vi "InterpretKeyboardCommand.vi"(6 "Key\nValue":i32, 8 "X Decreasing":string(combo)="10", 9 "X Increasing":string(combo)="13", 10 "Y Decreasing":string(combo)="28", 11 "Y Increasing":string(combo)="32") -> (0 "X Decreasing (#)":i32, 1 "X Increasing (#)":i32, 2 "Y Decreasing (#)":i32, 3 "Y Increasing (#)":i32, 4 "number":u32, 5 "Cluster of Input #s":cluster{i32, i32, i32, i32})   [LabVIEW 2011]
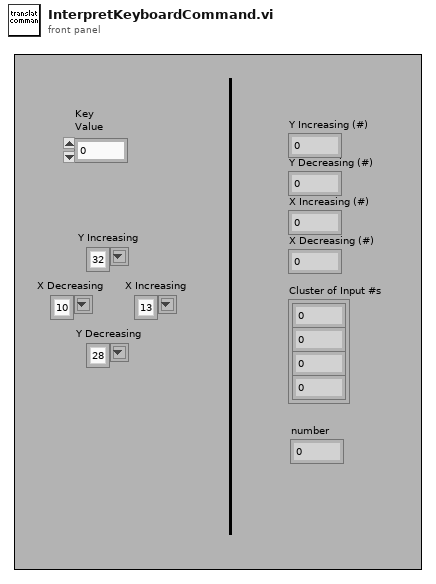
[diagram p1: front panel]
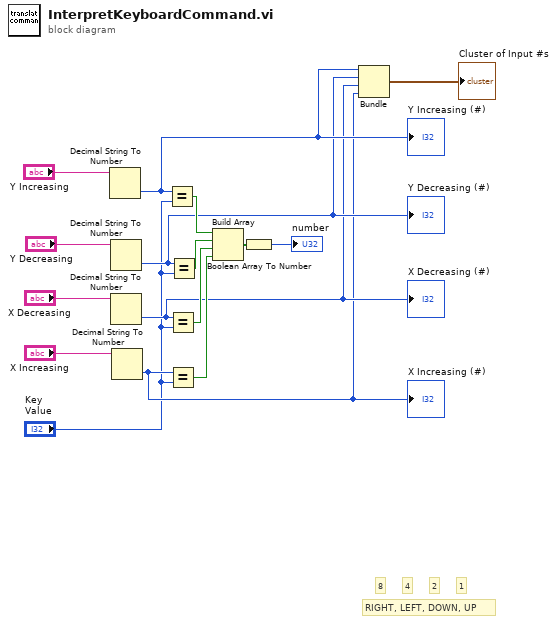
[diagram p0: block diagram]
diagram:
  # "8"
  # "4"
  # "2"
  # "1"
  # "RIGHT, LEFT, DOWN, UP"
  n1 = Decimal String To Number(string="Y Increasing") -> (number=w7:i32)  [unwired: 3 out]
  "Y Increasing (#)" <- w7
  n2 = Decimal String To Number(string="Y Decreasing") -> (number=w6:i32)  [unwired: 3 out]
  "Y Decreasing (#)" <- w6
  n3 = Decimal String To Number(string="X Decreasing") -> (number=w5:i32)  [unwired: 3 out]
  "X Decreasing (#)" <- w5
  n4 = Decimal String To Number(string="X Increasing") -> (number=w4:i32)  [unwired: 3 out]
  "X Increasing (#)" <- w4
  n5 = Equal?(x=w7, y="Key\nValue") -> (x = y?=w12:bool)
  n6 = Equal?(x=w5, y="Key\nValue") -> (x = y?=w10:bool)
  n7 = Equal?(x=w4, y="Key\nValue") -> (x = y?=w9:bool)
  n8 = Equal?(x=w6, y="Key\nValue") -> (x = y?=w11:bool)
  n9 = Build Array(w12, w11, w10, w9) -> (w8:bool[])
  n10 = Boolean Array To Number(Boolean array=w8) -> (number=→"number":u32)
  n11 = Bundle(w7, w6, w5, w4) -> (→"Cluster of Input #s":cluster{i32, i32, i32, i32})  [unwired: 1 out]
